vi "Verify With Regex Scrubber Count Unique Not Found.vi"(11 "LUnit Test Case In":refnum<class "Test Case.lvclass">) -> (0 "error out":errorcluster, 3 "LUnit Test Case Out":refnum<class "Test Case.lvclass">)   [LabVIEW 2020, in "Scrubber Tests.lvclass"]
uses:
  Scrubber Tests.lvclass
  <vilib>/Astemes/LUnit/Test Case.lvclass
  Source/Approval Tests/Regex Scrubber Count Unique/Regex Scrubber Count Unique.lvclass
  Source/Approval Tests/Options/Options.lvclass
  Source/Approval Tests/Scrubber/Scrubber.lvclass
  Source/Approval Tests/Namer/Namer.lvclass
  Source/Approval Tests/Naming Data/Naming Data.lvclass
  Source/Approval Tests/Reporter/Reporter.lvclass
  Source/Approval Tests/Text Comparator/Text Comparator.lvclass
  Scrubber Tests.lvclass/Scrubber Tests.ctl
  d22741b7-9abc-4f28-b51a-54e5e2d59af2.vi
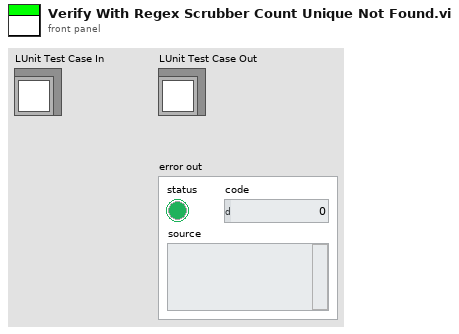
[diagram p1: front panel]
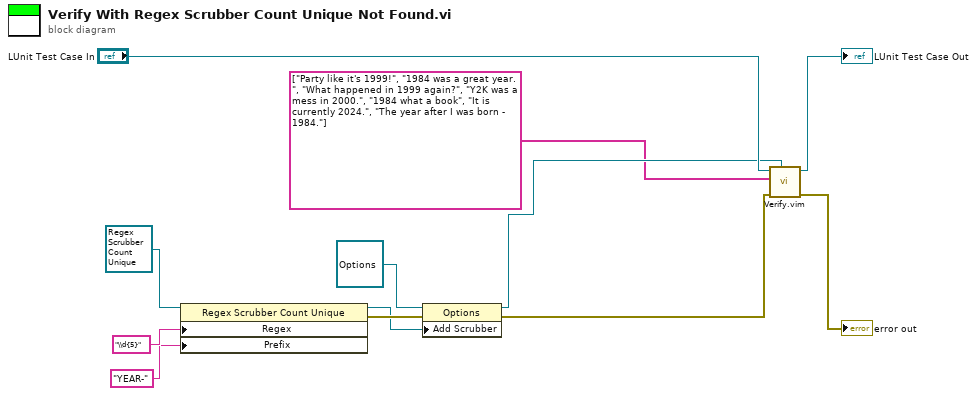
[diagram p0: block diagram]
diagram:
  n1 = property on="Property Node" class="Regex Scrubber Count Unique"(reference=refnum<class "Regex Scrubber Count Unique.lvclass"> refnum ("Approval Tests.lvlib:Regex Scrubber with Numbered Replacement.lvclass"), "Regex"="\\d{5}", "Prefix"="YEAR-" ("Replacement")) -> (reference out=w4:refnum<class "Regex Scrubber Count Unique.lvclass">, error out=w9:errorcluster)  [unwired: 1 in]
  n2 = property class="Options"(reference=refnum<class "Options.lvclass"> refnum ("Approval Tests.lvlib:Options.lvclass"), error in=w9, "Add Scrubber"=w4) -> (reference out=w2:refnum<class "Options.lvclass">, error out=w3:errorcluster)
  n3 = call "Verify.vim"("Options"=w2, "error in"=w3, "Test Data"=string[] ["Party like it's 1999!", "1984 was a great year.", "What happened in 1999 again?", "Y2K was a mess in 2000.", "1984 what a book", "It is currently 2024.", "The year after I was born - 1984."], "LUnit Test Case In"="LUnit Test Case In") -> ("error out"=→"error out":errorcluster, "LUnit Test Case Out"=→"LUnit Test Case Out":refnum<class "Test Case.lvclass">)  [unwired: 6 in]
